vi "update2D.vi"(8 "error in (no error)":errorcluster, 10 "reshapeInfo":T1, 11 "Image in":T4) -> (0 "error out":errorcluster, 3 "Image out":T4(plugin-control), 5 "time 2Dimage":u32)   [LabVIEW 2011, in "MagAnalysis_Online.lvclass"]
uses:
  MagAnalysis_Online.lvclass
  IMAQ Image.ctl
  reshapeINfo_TypDef.ctl
  emptyArray_TYpDEf.ctl
  emptyArrayCamX_TypDef.ctl
  NI_Vision_Development_Module.lvlib
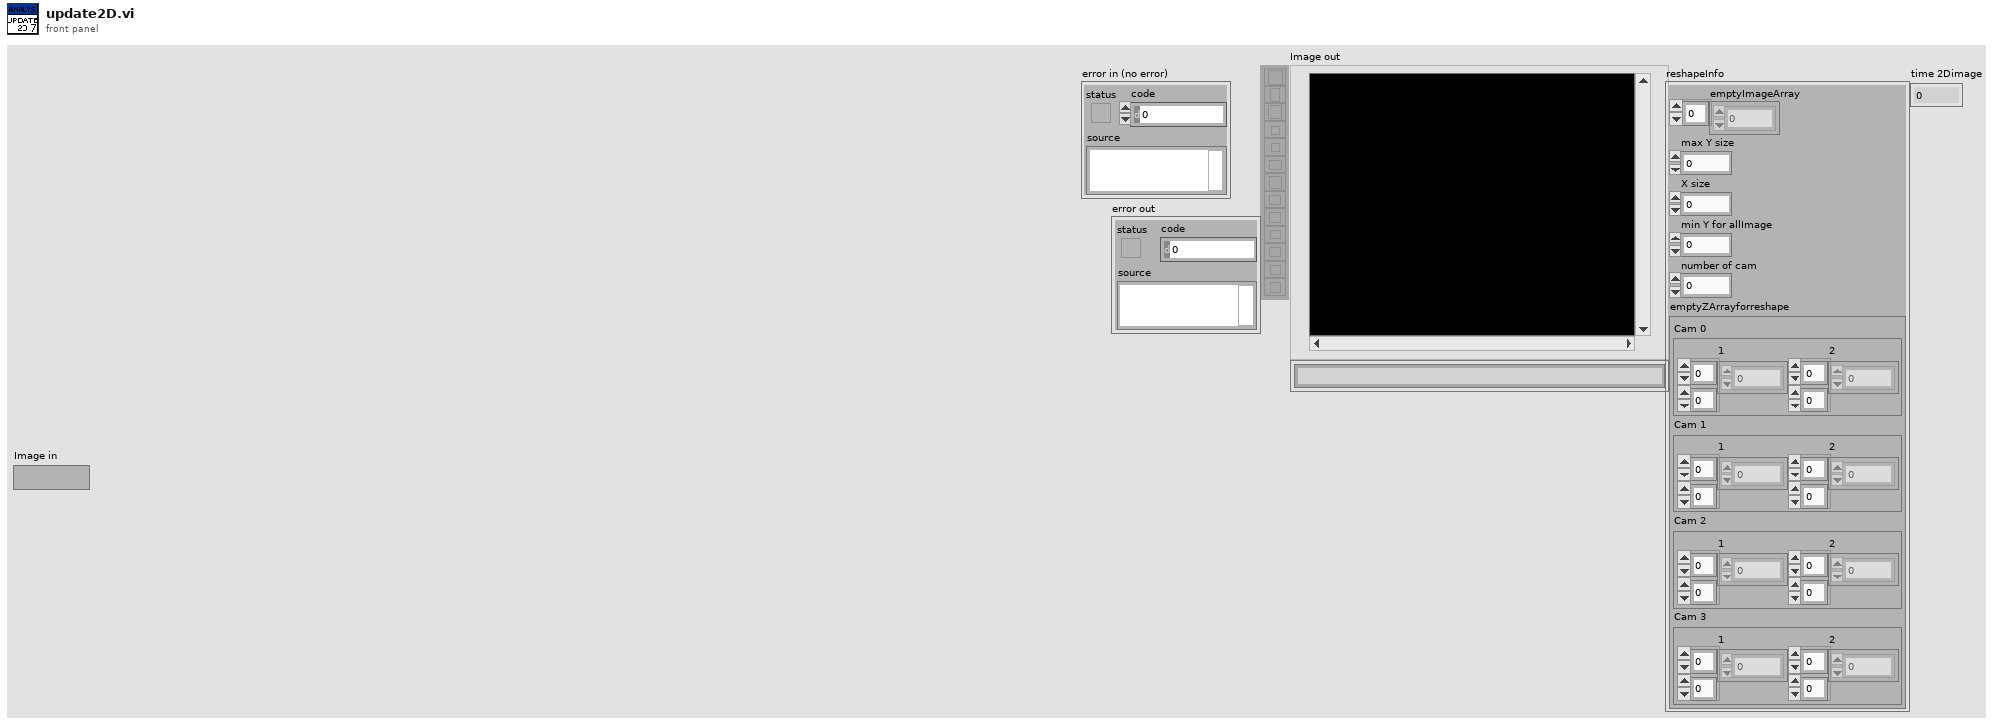
[diagram p1: front panel]
types:
  T1 = typedef "reshapeINfo_TypDef.ctl" = cluster{"emptyImageArray":dbl[], "max Y size":i32, "X size":i32, "min Y for allImage":dbl, "number of cam":i32, "emptyZArrayforreshape":T2}
  T2 = typedef "emptyArray_TYpDEf.ctl" = cluster{"Cam 0":T3, "Cam 1":T3, "Cam 2":T3, "Cam 3":T3}
  T3 = typedef "emptyArrayCamX_TypDef.ctl" = cluster{"1":dbl[][], "2":dbl[][]}
  T4 = typedef "IMAQ Image.ctl" = refnum<image>
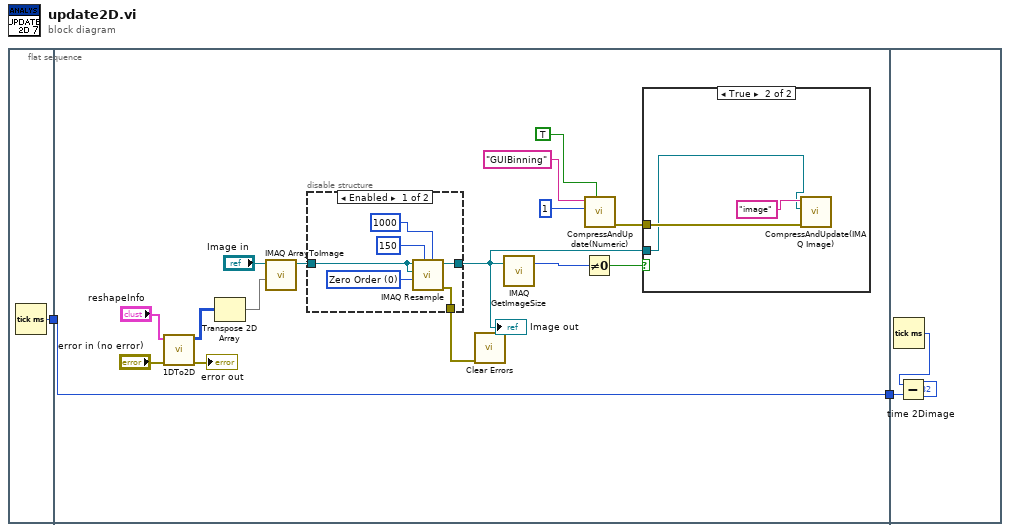
[diagram p0: block diagram]
diagram:
  n1 = flat-sequence {
    tunnel: [w3] -> w1
    tunnel: [w7] -> w2
    tunnel: w1 -> [w7]
    tunnel: w2 -> [w32]
    frame #0 {
      n2 = Tick Count (ms)() -> (millisecond timer value=w3:u32)
    }
    frame #1 {
      n3 = call "1DTo2D.vi"("error in (no error)"="error in (no error)", "reshapeInfo"="reshapeInfo") -> ("error in (no error) 2"=→"error out":errorcluster, "Array out"=w5:i16[][])  [unwired: 8 in]
      n4 = Transpose 2D Array(2D array=w5) -> (transposed array=w4:i16[][])
      n5 = call "IMAQ ArrayToImage"("Image Pixels (I16)"=w4, "Image"="Image in") -> ("Image Out"=w13:T4)  [unwired: 8 in, 1 out]
      n6 = disable-structure shown="Enabled" {
        disable-tunnel: w13 -> [w22 w26]
        disable-tunnel: [w21 w26] -> w11
        disable-tunnel: [w20 _] -> w6
        frame Enabled {
          w23 = u32 0 items=["Zero Order", "Bi-Linear", "Quadratic", "Cubic Spline"] ("Interpolation Type")
          n7 = call "IMAQ Resample"("X Resolution"=1000, "Y Resolution"=150, "Interpolation Type"=w23, "Image Dst"=w22, "Image Src"=w22) -> ("error out"=w20:errorcluster, "Image Dst Out"=w21:T4)  [unwired: 5 in]
        }
        frame Disabled {
        }
      }
      "Image out" <- w11
      n8 = call "Clear Errors.vi"("error in (no error)"=w6) -> ()  [unwired: 6 in, 1 out]
      n9 = call "IMAQ GetImageSize"("Image"=w11) -> ("Y Resolution"=w17:i32)  [unwired: 3 in, 2 out]
      n10 = Not Equal To 0?(x=w17) -> (x != 0?=w18:bool)
      n11 = call "CompressAndUpdate(Numeric).vi"("force CVT update (false)"=TRUE, "Numeric"=1, "command or variable name"="GUIBinning") -> ("error out"=w15:errorcluster)  [unwired: 8 in]
      n12 = case shown="True" w18 {
        tunnel: w15 -> [_ w29]
        tunnel: w11 -> [_ w27]
        frame False {
        }
        frame True {
          n13 = call "CompressAndUpdate(IMAQ Image).vi"("error in"=w29, "IMAQ Image"=w27, "command or variable name"="image") -> ()  [unwired: 8 in, 1 out]
        }
      }
    }
    frame #2 {
      n14 = Tick Count (ms)() -> (millisecond timer value=w31:u32)
      n15 = Subtract(x=w31, y=w32) -> (x-y=→"time 2Dimage":u32)
    }
  }
